vi "MM_PasteControls.vi"(6 "Position":T1, 8 "error in (no error)":errorcluster, 11 "vi ref in":refnum<vi>) -> (0 "error out":errorcluster, 2 "Controls":refnum<vi>[](array[refnum]), 3 "vi ref out":refnum<vi>)   [LabVIEW 2016]
uses:
  <vilib>/Utility/miscctls.llb/LVPositionTypeDef.ctl
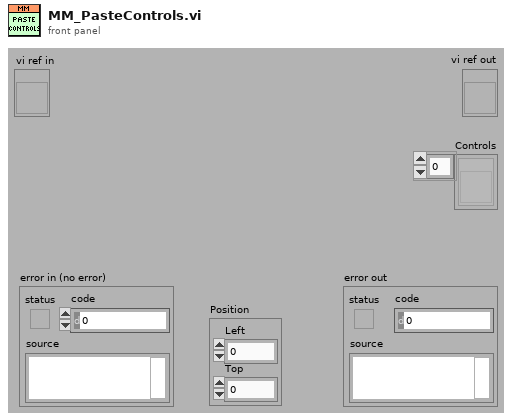
[diagram p1: front panel]
types:
  T1 = typedef "LVPositionTypeDef.ctl" = cluster{"Left":i32, "Top":i32}
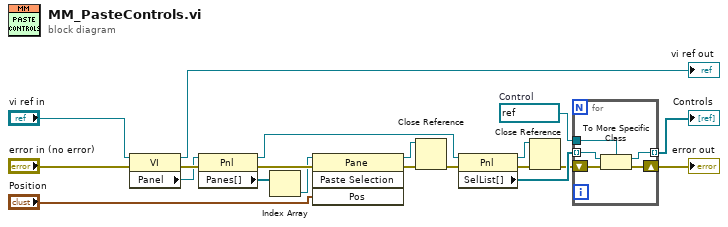
[diagram p0: block diagram]
diagram:
  w3 = refnum<vi> refnum  # Control
  n1 = property class="VI"(reference="vi ref in", error in="error in (no error)") -> (reference out=→"vi ref out":refnum<vi>, error out=w8:errorcluster, "Panel"=w7:refnum<vi>)
  n2 = property class="Pnl"(reference=w7, error in=w8) -> (reference out=w16:refnum<vi>, error out=w9:errorcluster, "Panes[]"=w5:refnum<vi>[])
  n3 = Index Array(array=w5) -> (element=w6:refnum<vi>)  [unwired: 1 in]
  n4 = invoke class="Pane" method="Paste Selection"(reference=w6, error in=w9, "Pos"="Position") -> (reference out=w15:refnum<vi>, error out=w14:errorcluster)  [unwired: 1 in, 2 out]
  n5 = Close Reference(reference=w15, error in (no error)=w14) -> (error out=w17:errorcluster)
  n6 = property class="Pnl"(reference=w16, error in=w17) -> (reference out=w18:refnum<vi>, error out=w19:errorcluster, "SelList[]"=w20:refnum<vi>[])
  n7 = Close Reference(reference=w18, error in (no error)=w19) -> (error out=w2:errorcluster)
  n8 = for {
    tunnel: w20 -> [w25] mode=indexing
    tunnel: [w24] -> w4 mode=indexing
    tunnel: w3 -> [w21]
    shift-right: [w22] -> w1
    shift-left: w2 -> [w23]
    n9 = To More Specific Class(target class=w21, reference=w25, error in=w23) -> (specific class reference=w24:refnum<vi>, error out=w22:errorcluster)
  }
  "Controls" <- w4
  "error out" <- w1
